vi "StartSerial.vi"(8 "error in":errorcluster, 9 "baud rate":u32=115200, 11 "VISA Refnum in":refnum<visa-resource-name>) -> (0 "error out":errorcluster, 3 "VISA Refnum out":refnum<visa-resource-name>)   [LabVIEW 2014, in "Manipulator.lvclass"]
uses:
  Manipulator.lvclass
  <vilib>/Instr/_visa.llb/VISA Configure Serial Port (Instr).vi
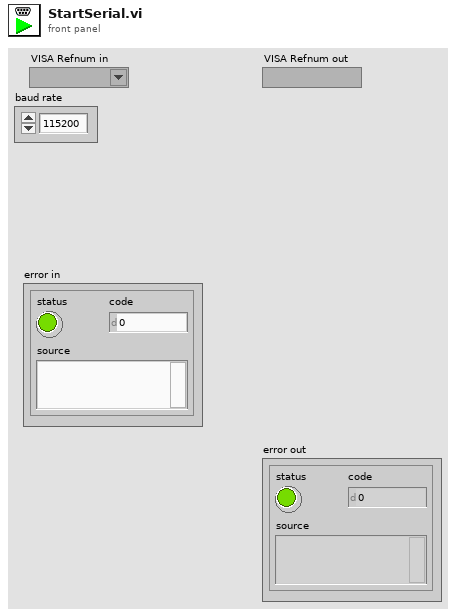
[diagram p1: front panel]
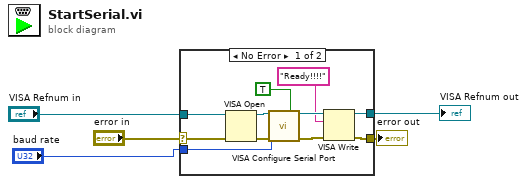
[diagram p0: block diagram]
diagram:
  n1 = case shown="No Error" "error in" {
    selector: "error in" -> [w13 w18]
    tunnel: [w7 w18] -> w5
    tunnel: "VISA Refnum in" -> [w16 w17]
    tunnel: [w9 w17] -> w3
    tunnel: "baud rate" -> [w11 _]
    frame No Error {
      n2 = VISA Open(error in (no error)=w13, VISA resource name=w16) -> (VISA resource name=w14:refnum<visa-resource-name>, error out=w15:errorcluster)  [unwired: 3 in]
      n3 = call-poly "VISA Configure Serial Port"("VISA resource name"=w14, "Enable Termination\nChar (T)"=TRUE ("Enable Termination\nChar (T)"), "baud rate (9600)"=w11, "error in (no error)"=w15) -> ("VISA resource name out"=w10:refnum<visa-resource-name>, "error out"=w8:errorcluster)  [unwired: 10 in]
      n4 = VISA Write(VISA resource name=w10, write buffer="Ready!!!!", error in (no error)=w8) -> (VISA resource name out=w9:refnum<visa-resource-name>, error out=w7:errorcluster)  [unwired: 1 out]
    }
    frame Error {
    }
  }
  "error out" <- w5
  "VISA Refnum out" <- w3
